vi "mainVItestt.vi"() -> ()   [LabVIEW 2017]
uses:
  Controls/DataCluster.ctl
panel:
  out "I":dbl
  out "e":dbl
  out "output variable":dbl
  out "CV":dbl
  in  "TD":dbl
  in  "TI":dbl
  in  "kr":dbl
  in  "SP":dbl
  out "Waveform Chart":cluster{"P1":dbl, "P2":dbl, "P3":dbl}(graph)
  in  "NIS":u32
  in  "Dt":u32
  in  "Stop Button":bool
  out "P0":dbl(slide) scale=0.0..10.0 scale format="%#_6p"
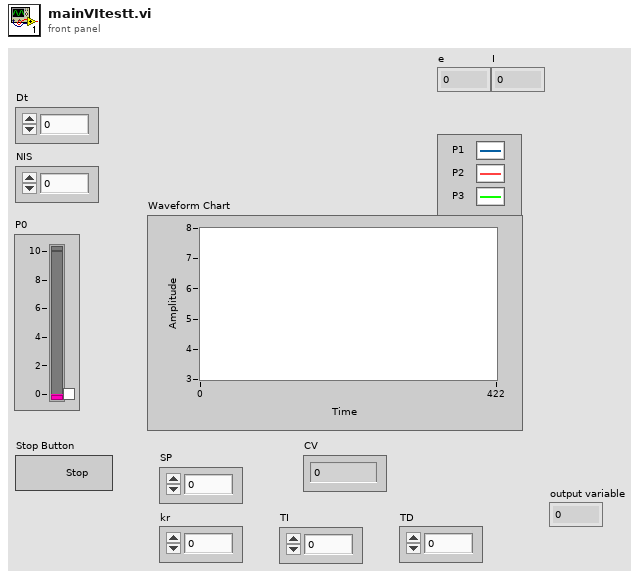
[diagram p1: front panel]
types:
  T1 = enum16{"open", "replace", "create", "open or create", "replace or create", "replace or create with confirmation"}
  T2 = typedef "DataCluster.ctl" = cluster{"P1":dbl, "P2":dbl, "P3":dbl}
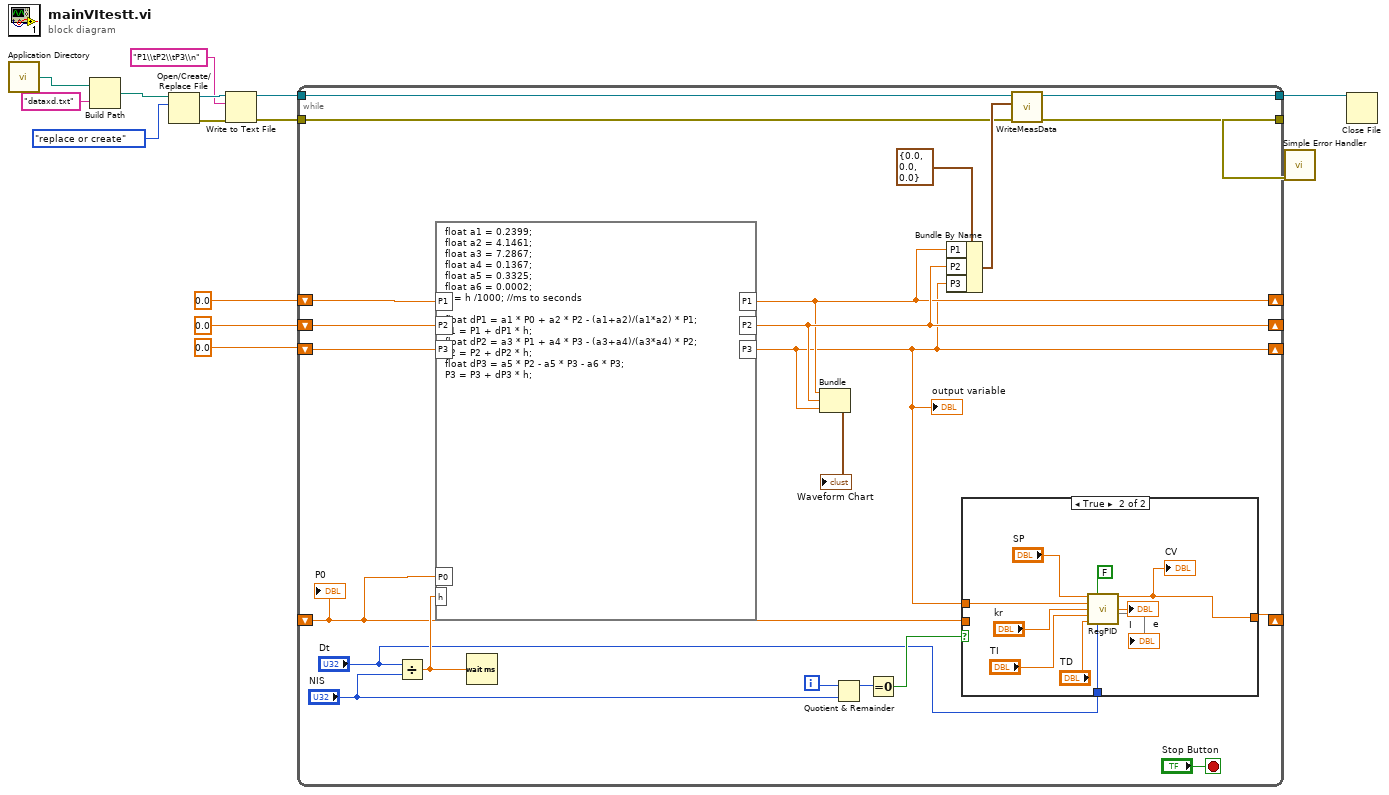
[diagram p0: block diagram]
diagram:
  n1 = call <vilib>:"Application Directory.vi"() -> ("Application Directory"=w9:path)
  n2 = Build Path(base path=w9, name or relative path="dataxd.txt") -> (appended path=w8:path)
  n3 = Open/Create/Replace File(file path (use dialog)=w8, operation (0:open)=T1."replace or create") -> (refnum out=w5:refnum<file>, error out=w2:errorcluster)  [unwired: 4 in, 1 out]
  n4 = Write to Text File(file (use dialog)=w5, text="P1\\tP2\\tP3\\n", error in=w2) -> (refnum out=w4:refnum<file>, error out=w3:errorcluster)  [unwired: 1 in, 1 out]
  n5 = while {
    shift-right: [w25] -> _
    shift-left: 0.0 -> [w36]
    shift-right: [w26] -> _
    shift-left: 0.0 -> [w35]
    shift-right: [w19] -> _
    shift-left: 0.0 -> [w34]
    tunnel: w4 -> [w31]
    tunnel: [w30] -> w10
    tunnel: w3 -> [w28]
    tunnel: [w27] -> w6
    shift-right: [w18] -> _
    shift-left: _ -> [w16]
    i -> [w23]
    stop <- "Stop Button" stop-if-true
    n6 = Divide(x="Dt", y="NIS") -> (x/y=w17:dbl)
    n7 = formula code="float a1 = 0.2399;\nfloat a2 = 4.1461;\nfloat a3 = 7.2867;\nfloat a4 = 0.1367;\nfloat a5 = 0.3325;\nfloat a6 = 0.0002;\nh = h /1000; //ms to seconds\n\nfloat dP1 = a1 * P0 + a2 * P2 - (a1+a2)/(a1*a2) * P1;\nP1 = P1 + dP1 * h;\nfloat dP2 = a3 * P1 + a4 * P3 - (a3+a4)/(a3*a4) * P2;\nP2 = P2 + dP2 * h;\nfloat dP3 = a5 * P2 - a5 * P3 - a6 * P3;\nP3 = P3 + dP3 * h;"("P0"=w16, "P1"=w36, "P2"=w35, "P3"=w34, "h"=w17) -> ("P1"=w25:dbl, "P2"=w26:dbl, "P3"=w19:dbl)
    "output variable" <- w19
    n8 = Wait (ms)(milliseconds to wait=w17) -> ()  [unwired: 1 out]
    n9 = Bundle("P1"=w25, "P2"=w26, "P3"=w19) -> (→"Waveform Chart":cluster{"P1":dbl, "P2":dbl, "P3":dbl})  [unwired: 1 in]
    n10 = Quotient & Remainder(x=w23, y="NIS") -> (x-y*floor(x/y)=w21:u32)  [unwired: 1 out]
    n11 = Equal To 0?(x=w21) -> (x = 0?=w20:bool)
    n12 = Bundle By Name(cluster=T2 {"P1"=0.0, "P2"=0.0, "P3"=0.0} ("Cluster"), "P1"=w25, "P2"=w26, "P3"=w19) -> (w29:T2)
    n13 = case shown="True" w20 {
      tunnel: w19 -> [_ w46]
      tunnel: "Dt" -> [_ w41]
      tunnel: [w37 w40] -> w18
      tunnel: w16 -> [w37 _]
      frame False {
      }
      frame True {
        n14 = call "RegPID.vi"("SP"="SP", "init"=FALSE, "PV"=w46, "kr"="kr", "TI"="TI", "TD"="TD", "h"=w41) -> ("CV"=w40:dbl, "e"=→"e":dbl, 15:→"I")  [unwired: 6 in]
        "CV" <- w40
      }
    }
    n15 = call "WriteMeasData.vi"("error in (no error)"=w28, "Data Cluster"=w29, "Byte Stream File in"=w31) -> ("error out"=w27:errorcluster, "Byte Stream File out"=w30:refnum<file>)  [unwired: 7 in]
    "P0" <- w16
  }
  n16 = call <vilib>:"Simple Error Handler.vi"("error in (no error)"=w6) -> ()  [unwired: 4 in, 5 out]
  n17 = Close File(refnum=w10) -> ()  [unwired: 1 in, 2 out]
